vi "GetMatchedString.vi"(10 "パターン文字列":string, 11 "探索配列":string[](array[string])) -> (3 "一致配列":string[](array[string]))   [LabVIEW 2015]
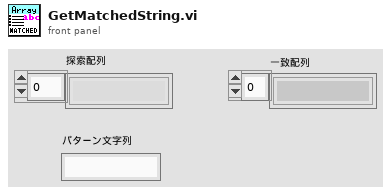
[diagram p1: front panel]
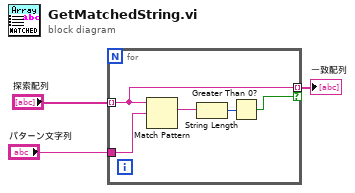
[diagram p0: block diagram]
diagram:
  n1 = for {
    tunnel: "探索配列" -> [w5] mode=indexing
    tunnel: "パターン文字列" -> [w8]
    tunnel: [w5] -> w1 mode=indexing if=w4
    n2 = Match Pattern(string=w5, regular expression=w8) -> (match substring=w7:string)  [unwired: 1 in, 3 out]
    n3 = String Length(string=w7) -> (length=w6:i32)
    n4 = Greater Than 0?(x=w6) -> (x > 0?=w4:bool)
  }
  "一致配列" <- w1
